vi "Remove VI filetype extension.vi"(8 "Error In":errorcluster, 11 "VI name IN":string) -> (0 "Error Out":errorcluster, 3 "Trimmed name OUT":string)   [LabVIEW 2012]
doc: "SciScan 1.2 160622\nThis VI removes the '.vi' extension from the input VI name string"
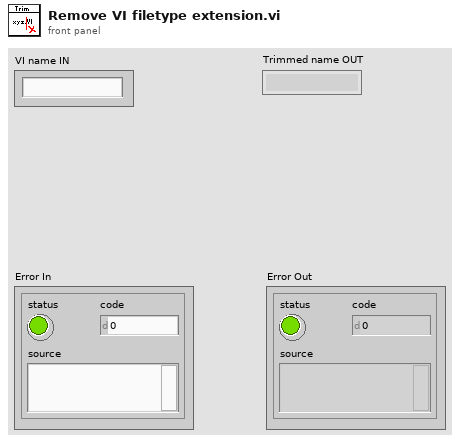
[diagram p1: front panel]
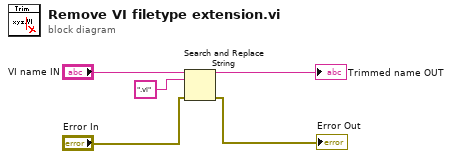
[diagram p0: block diagram]
diagram:
  n1 = Search and Replace String(input string="VI name IN", search string=".vi", error in="Error In") -> (result string=→"Trimmed name OUT":string, error out=→"Error Out":errorcluster)  [unwired: 5 in, 2 out]
